vi "Event-Acquisition-mode.vi"(7 "Acquis. mode":T1(ring), 8 "error in (no error)":errorcluster, 10 "Data ref. in":refnum<data-value>, 11 "UI ref. in":refnum<data-value>) -> (0 "error out":errorcluster, 2 "Data ref.":refnum<data-value>, 3 "UI ref.":refnum<data-value>)   [LabVIEW 2013, in "CameraVision.lvlib" / "CV-UI.lvclass"]
uses:
  CV-UI.lvclass
  Main/CV-Main.lvclass
  Control-names.ctl
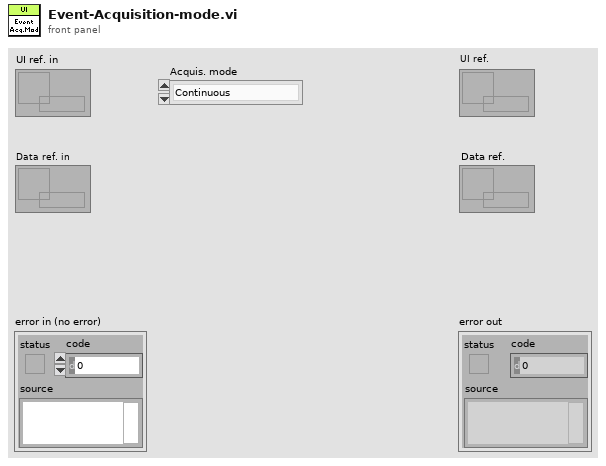
[diagram p1: front panel]
types:
  T1 = enum16{"Continuous", "Continuous batch", "Single batch", "Single batch -delayed"}
  T2 = typedef "CameraVision.lvlib/CV-UI.lvclass/Control-names.ctl" = enum16{"Start acquisition", "Activate", "Stop acquisition", "Settings type", "Load settings", "Save settings", "Import images", "Camera selector", "Image type selector", "Batch browser", "Image refresh", "Parameter tabs", "Displays", "Processing tabs", "Processing selector", "Map characteristic", "Show info", "Manual trigger"}
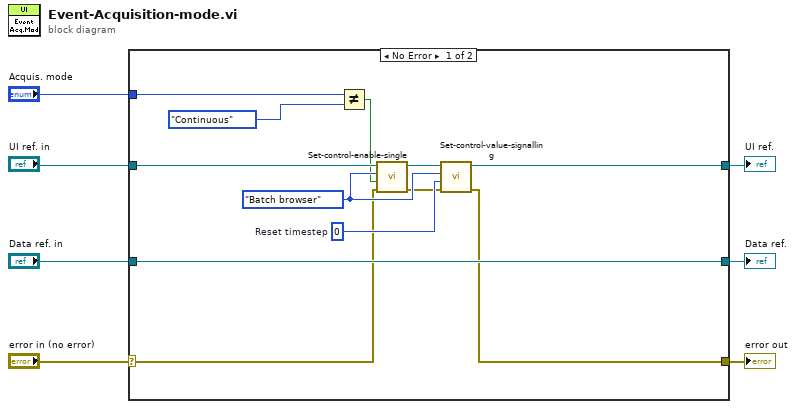
[diagram p0: block diagram]
diagram:
  n1 = case shown="No Error" "error in (no error)" {
    selector: "error in (no error)" -> [w9 w22]
    tunnel: [w8 w22] -> w6
    tunnel: [w12 w21] -> w4
    tunnel: "UI ref. in" -> [w14 w21]
    tunnel: "Data ref. in" -> [w19 w20]
    tunnel: "Acquis. mode" -> [w18 _]
    tunnel: [w19 w20] -> w2
    frame No Error {
      w15 = Control-names."Batch browser" ("Control name")
      w16 = 0  # Reset timestep
      n2 = Not Equal?(x=w18, y=T1."Continuous") -> (x != y?=w11:bool)
      n3 = call "Set-control-enable-single.vi"("error in (no error)"=w9, "Enable?"=w11, "Control name"=w15, "UI ref. in"=w14) -> ("error out"=w10:errorcluster, "UI ref."=w13:refnum<data-value>)  [unwired: 6 in]
      n4 = call "Set-control-value-signalling.vi"("error in (no error)"=w10, "Value"=w16, "Control name"=w15, "UI ref. in"=w13) -> ("error out"=w8:errorcluster, "UI ref."=w12:refnum<data-value>)  [unwired: 6 in]
    }
    frame Error {
    }
  }
  "error out" <- w6
  "Data ref." <- w2
  "UI ref." <- w4
